vi "Get Detail.vi"(11 "ErrorOrSuccess JSON in":refnum<class "ErrorOrSuccess JSON.lvclass">) -> (2 "Error/Abort details (JSON)":T1={"Error URI"="", "Error Arguments"="[]", "Error ArgumentKw"="{}", "Error Details"="{}", "Associated LabVIEW Error"={"status"=FALSE, "code"=0, "source"=""}}, 3 "ErrorOrSuccess JSON out":refnum<class "ErrorOrSuccess JSON.lvclass">)   [LabVIEW 2020, in "wamplv.lvlib" / "ErrorOrSuccess JSON.lvclass"]
uses:
  ErrorOrSuccess JSON.lvclass
  ErrorOrSuccess JSON.lvclass/ErrorOrSuccess JSON.ctl
  WAMP Client/API/TypeDefs/Error or abort detail (JSON).ctl
  wamplv.lvlib
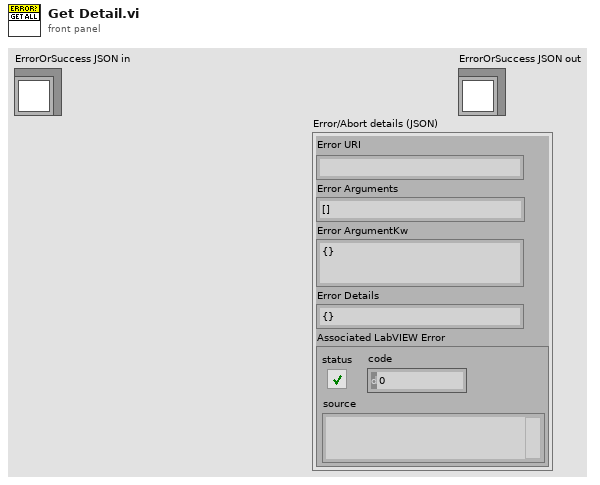
[diagram p1: front panel]
types:
  T1 = typedef "wamplv.lvlib/Error or abort detail (JSON).ctl" = cluster{"Error URI":string, "Error Arguments":string, "Error ArgumentKw":string, "Error Details":string, "Associated LabVIEW Error":errorcluster}
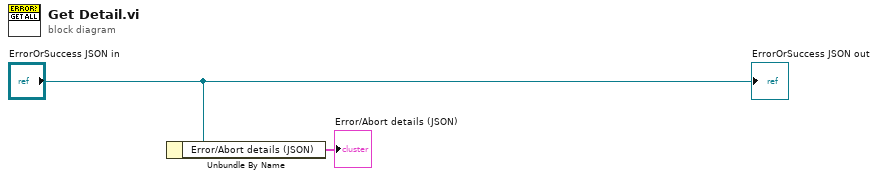
[diagram p0: block diagram]
diagram:
  n1 = Unbundle By Name("ErrorOrSuccess JSON in") -> ("Error/Abort details (JSON)"=→"Error/Abort details (JSON)":T1)
  "ErrorOrSuccess JSON out" <- "ErrorOrSuccess JSON in"
